vi "gun_tracking_data_store.vi"(10 "Mode":enum16{"Set", "Get"}(ring), 11 "Compound Target Data":T2) -> (2 "New Data":bool, 3 "Compound Target Data Out":T2)   [LabVIEW 2011]
uses:
  2012vision/Camera State.ctl
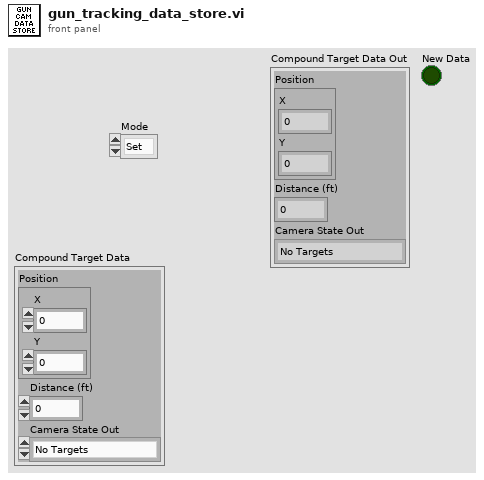
[diagram p1: front panel]
types:
  T1 = typedef "Camera State.ctl" = enum16{"No Targets", "Low Confidence", "Medium Confidence", "High Confidence", "Camera Error"}
  T2 = cluster{"Position":cluster{"X":dbl, "Y":dbl}, "Distance (ft)":dbl, "Camera State Out":T1}
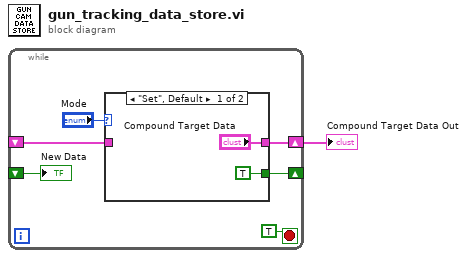
[diagram p0: block diagram]
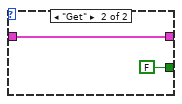
[diagram p2: hidden frame]
diagram:
  n1 = while {
    shift-right: [w5] -> w1
    shift-left: _ -> [w4]
    shift-right: [w3] -> _
    shift-left: _ -> [w2]
    stop <- TRUE stop-if-true
    n2 = case shown="\"Set\", Default" "Mode" {
      tunnel: ["Compound Target Data" w11] -> w5
      tunnel: w4 -> [_ w11]
      tunnel: [TRUE FALSE] -> w3
      frame "Set", Default {
      }
      frame "Get" {
      }
    }
    "New Data" <- w2
  }
  "Compound Target Data Out" <- w1
